vi "Pulse Stretch Demonstrator.vi"() -> ()   [LabVIEW 2011]
panel:
  out "Stretch Out":bool
  in  "Stretch (sec)":dbl=1.0
  in  "input":bool
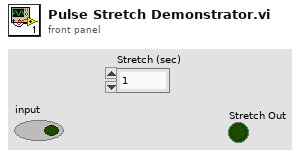
[diagram p1: front panel]
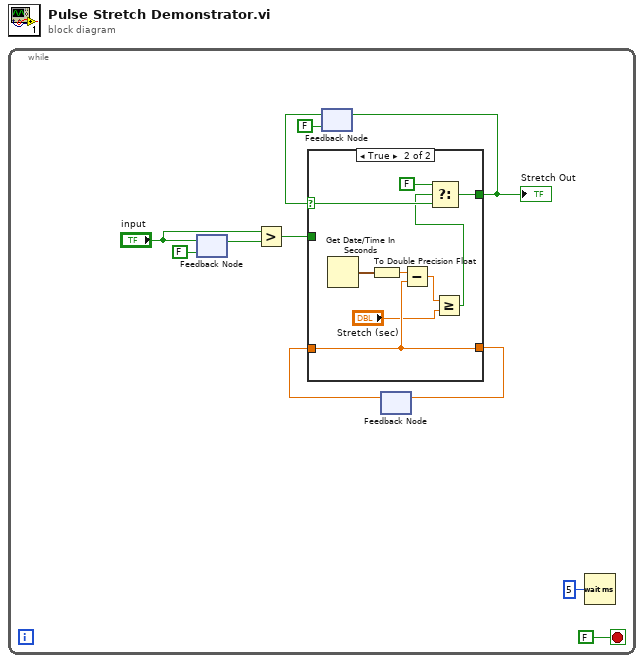
[diagram p0: block diagram]
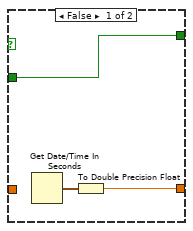
[diagram p2: hidden frame]
diagram:
  n1 = while {
    stop <- FALSE stop-if-true
    n2 = feedback-in #1("input") -> ()
    n3 = feedback #1(FALSE ("input")) -> (w8:bool)
    n4 = Greater?(x="input", y=w8) -> (0:w1:bool)
    n5 = feedback #2(FALSE) -> (w3:bool)
    n6 = feedback #3() -> (w5:dbl)  [unwired: 1 in]
    n7 = case shown="True" w3 {
      selector: w3 -> [_ w18]
      tunnel: [w13 w21] -> w6
      tunnel: w5 -> [_ w21]
      tunnel: [w12 w16] -> w4
      tunnel: w1 -> [w12 _]
      frame False {
        n8 = Get Date/Time In Seconds() -> (seconds since 1Jan1904=w14:timestamp)
        n9 = To Double Precision Float(number=w14) -> (double precision float=w13:dbl)
      }
      frame True {
        n10 = Get Date/Time In Seconds() -> (seconds since 1Jan1904=w23:timestamp)
        n11 = To Double Precision Float(number=w23) -> (double precision float=w22:dbl)
        n12 = Subtract(x=w22, y=w21) -> (x-y=w20:dbl)
        n13 = Greater Or Equal?(x=w20, y="Stretch (sec)") -> (x >= y?=w17:bool)
        n14 = Select(t=FALSE, s=w17, f=w18) -> (s? t:f=w16:bool)
      }
    }
    "Stretch Out" <- w4
    n15 = feedback-in #2(w4) -> ()
    n16 = feedback-in #3(w6) -> ()
    n17 = Wait (ms)(milliseconds to wait=u32 5) -> ()  [unwired: 1 out]
  }
